vi "Mark Implementor In Tree.vi"(2 "error in (no error)":errorcluster, 3 "Item ID to mark":string, 4 "Tree Refnum in":refnum<vi>) -> (0 "error out":errorcluster, 1 "Tree Refnum out":refnum<vi>)   [LabVIEW 2020, in "Choose Implementation Dialog.lvlib"]
uses:
  Choose Implementation Dialog.lvlib
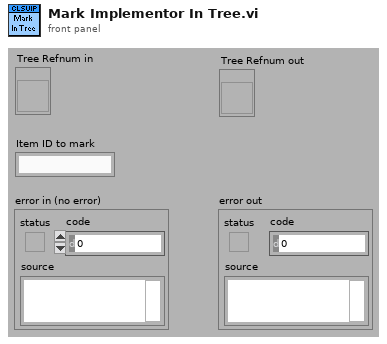
[diagram p1: front panel]
types:
  T1 = typedef "imagedata.ctl" = cluster{"image type":i32, "image depth":i32, "image":u8[], "mask":u8[], "colors":u32[], "Rectangle":cluster{"left":i16, "top":i16, "right":i16, "bottom":i16}}
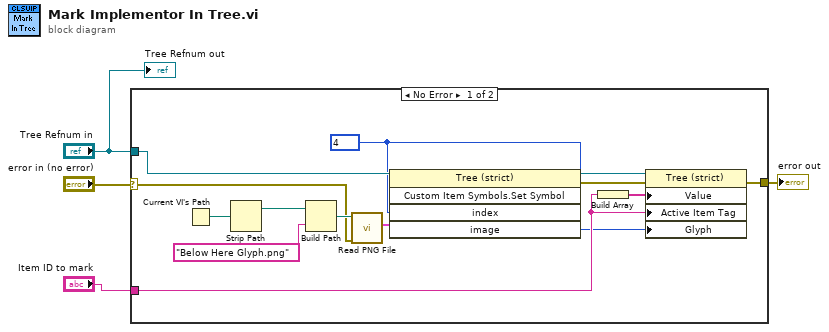
[diagram p0: block diagram]
diagram:
  n1 = case shown="No Error" "error in (no error)" {
    selector: "error in (no error)" -> [w8 w18]
    tunnel: [w16 w18] -> w4
    tunnel: "Tree Refnum in" -> [w10 _]
    tunnel: "Item ID to mark" -> [w9 _]
    frame No Error {
      w5 = 4
      n2 = Current VI's Path() -> (path=w14:path)
      n3 = Strip Path(path=w14) -> (stripped path=w13:path)  [unwired: 1 out]
      n4 = Build Path(base path=w13, name or relative path="Below Here Glyph.png") -> (appended path=w11:path)
      n5 = call <vilib>:"Read PNG File.vi"("error in (no error)"=w8, "path to PNG file"=w11) -> ("image data"=w15:T1)  [unwired: 7 in, 2 out]
      n6 = invoke class="Tree (strict)" method="Custom Item Symbols.Set Symbol"(reference=w10, "index"=w5, "image"=w15) -> (reference out=w7:refnum<vi>, error out=w6:errorcluster)  [unwired: 2 in, 3 out]
      n7 = Build Array(w9) -> (w17:string[])
      n8 = property class="Tree (strict)"(reference=w7, error in=w6, "Value"=w17, "Active Item Tag"=w9, "Glyph"=w5) -> (error out=w16:errorcluster)  [unwired: 1 out]
    }
    frame Error {
    }
  }
  "error out" <- w4
  "Tree Refnum out" <- "Tree Refnum in"
